vi "ReadHeader.vi"(2 "Filename":string, 3 "NXT":T1={"Hardware"="NXT", "Flattened String"=""}) -> (0 "NXT":T1={"Hardware"="NXT", "Flattened String"=""})   [LabVIEW 2010, in "Packet Recorder.lvlib"]
uses:
  Packet Recorder.lvlib
  <vilib>/NXT/Subs/LVHSConnector.ctl
  Components/Components.llb/Integer to Boolean Array_U16.vi
  Components/Components.llb/Integer to Boolean Array_U32.vi
  Components/Components.lvlib
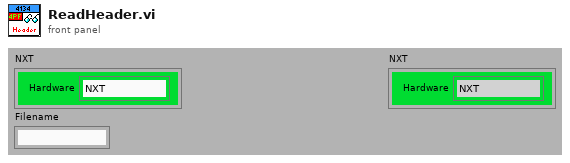
[diagram p1: front panel]
types:
  T1 = typedef "LVHSConnector.ctl" = cluster{"Hardware":string, "Flattened String":string}
  T2 = enum16{"big-endian, network order", "native, host order", "little-endian"}
  T3 = cluster{"Boolean array":bool[], "Boolean array":bool[]}
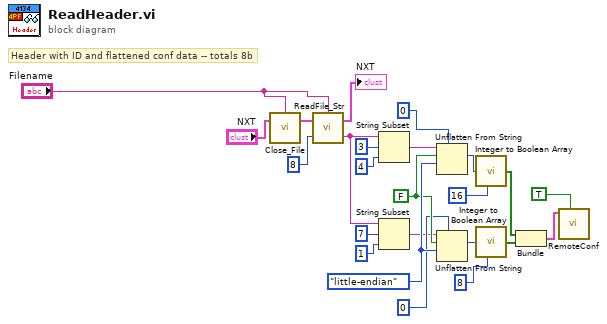
[diagram p0: block diagram]
diagram:
  w13 = FALSE ("data includes array or string size? (T)")
  w14 = T2."little-endian" ("byte order (0:big-endian, network order)")
  # "Header with ID and flattened conf data -- totals 8b"
  n1 = call <vilib>:"Close_File.vi"("NXT"="NXT", "Filename"="Filename") -> ("NXT"=w1:T1)  [unwired: 2 in]
  n2 = call <vilib>:"ReadFile_Str.vi"("Length (1)"=u32 8, "NXT"=w1, "Filename"="Filename") -> ("String"=w20:string, "NXT"=→"NXT":T1)
  n3 = String Subset(string=w20, offset (0)=3, length (rest)=4 ("length (rest)")) -> (substring=w19:string)
  n4 = String Subset(string=w20, offset (0)=7, length (rest)=1 ("length (rest)")) -> (substring=w11:string)
  n5 = Unflatten From String(type=u32 0 ("unsigned 8bit integer"), binary string=w19, data includes array or string size? (T)=w13, byte order (0:big-endian, network order)=w14) -> (value=w4:u32)  [unwired: 1 in, 2 out]
  n6 = Unflatten From String(type=u8 0 ("unsigned 8bit integer"), binary string=w11, data includes array or string size? (T)=w13, byte order (0:big-endian, network order)=w14) -> (value=w9:u8)  [unwired: 1 in, 2 out]
  n7 = call-poly "Integer to Boolean Array.vi"("number"=w4, "minimum"=u32 16) -> ("Boolean array"=w5:bool[])  [unwired: 5 in]
  n8 = call-poly "Integer to Boolean Array.vi"("number"=w9, "minimum"=u32 8) -> ("Boolean array"=w8:bool[])  [unwired: 5 in]
  n9 = Bundle("Boolean array"=w5, "Boolean array"=w8) -> (w16:T3)  [unwired: 1 in]
  n10 = call "RemoteConf.vi"("Write?"=TRUE, "ConfInput"=w16) -> ()  [unwired: 9 in, 1 out]
